vi "Send Message.vi"(6 "ID":string, 8 "error in (no error)":errorcluster, 9 "Data":variant, 10 "Command":string, 11 "RemoteControl.ZMQ in":refnum<class "RemoteControl.ZMQ.lvclass">) -> (0 "error out":errorcluster, 3 "RemoteControl.ZMQ out":refnum<class "RemoteControl.ZMQ.lvclass">)   [LabVIEW 2019, in "RemoteControl.ZMQ.lvlib" / "RemoteControl.ZMQ.lvclass"]
uses:
  RemoteControl.ZMQ.lvclass
  C:/Program Files (x86)/National Instruments/LabVIEW 2019/user.lib/LevyLab/RemoteControl/RemoteControl/RemoteControl.lvclass
  RemoteControl.ZMQ.lvclass/RemoteControl.ZMQ.ctl
  <userlib>/LevyLab/RemoteControl/RemoteControl/RemoteControl.lvclass/RemoteControl.ctl
  <vilib>/PRIrvin/JSON-RPC/JSON-RPC.lvlib
  <vilib>/addons/zeromq/zmq_socket.lvclass
  <userlib>/LevyLab/RemoteControl/RemoteControl/RemoteControl.lvclass
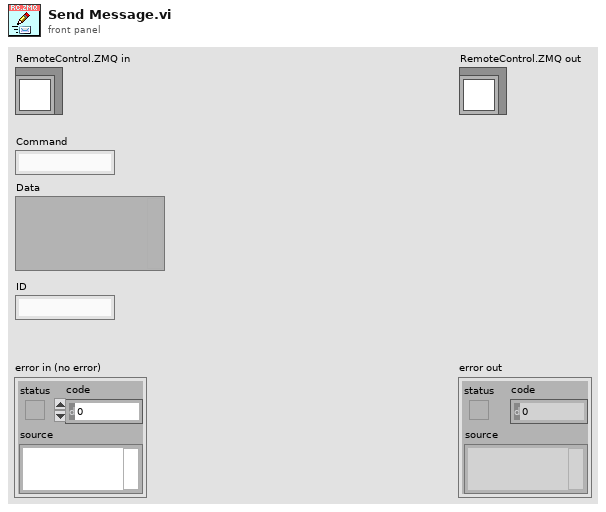
[diagram p1: front panel]
types:
  T1 = typedef "zeromq.lvlib/socket_type.ctl" = enum8{"ZMQ_PAIR", "ZMQ_PUB", "ZMQ_SUB", "ZMQ_REQ", "ZMQ_REP", "ZMQ_DEALER", "ZMQ_ROUTER", "ZMQ_PULL", "ZMQ_PUSH", "ZMQ_XPUB", "ZMQ_XSUB", "ZMQ_STREAM", "ZMQ_SERVER", "ZMQ_CLIENT", "ZMQ_RADIO", "ZMQ_DISH", "ZMQ_GATHER", "ZMQ_SCATTER", "ZMQ_DGRAM"}
  T2 = cluster{"Command":string, "Data":variant, "ID":string}
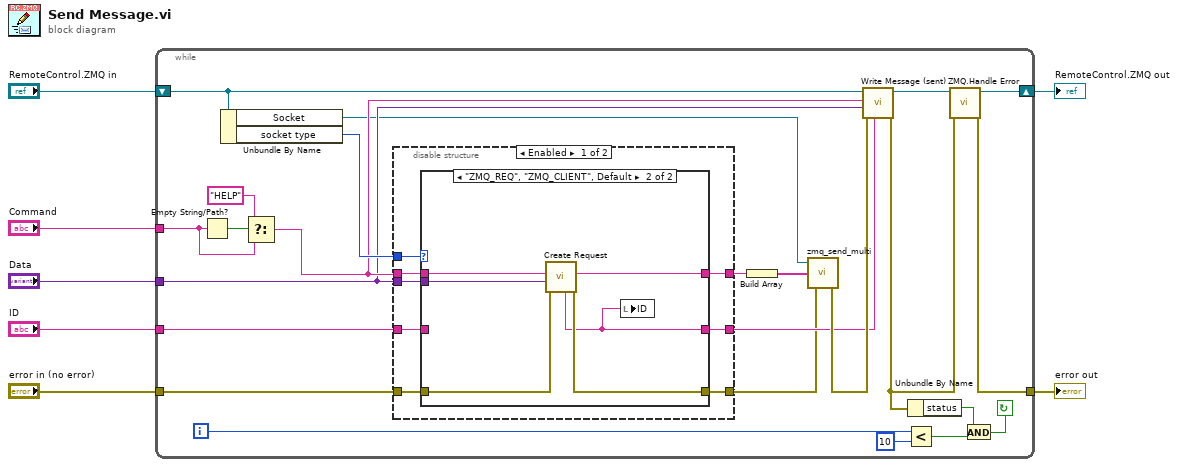
[diagram p0: block diagram]
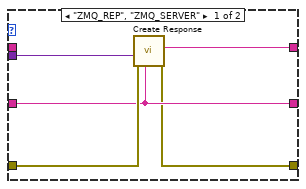
[diagram p2: hidden frame]
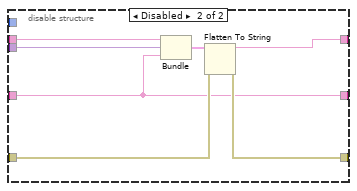
[diagram p3: hidden frame]
diagram:
  n1 = while {
    tunnel: "Command" -> [w15]
    tunnel: "ID" -> [w28]
    tunnel: "Data" -> [w23]
    shift-right: [w17] -> w4
    shift-left: "RemoteControl.ZMQ in" -> [w19]
    tunnel: "error in (no error)" -> [w8]
    tunnel: [w16] -> w3
    i -> [w14]
    stop <- w11 continue-if-true
    n2 = Empty String/Path?(string/path=w15) -> (empty?=w30:bool)
    n3 = Unbundle By Name(w19) -> ("Socket"=w22:refnum<class "zmq_socket.lvclass">, "socket type"=w29:T1)
    n4 = Select(t="HELP", s=w30, f=w15) -> (s? t:f=w27:string)
    n5 = disable-structure shown="Enabled" {
      disable-tunnel: w23 -> [w39 w53]
      disable-tunnel: w27 -> [w38 w54]
      disable-tunnel: [w37 w51] -> w24
      disable-tunnel: w8 -> [w36 w56]
      disable-tunnel: [w35 w55] -> w20
      disable-tunnel: w29 -> [w34 _]
      disable-tunnel: w28 -> [w32 w52]
      disable-tunnel: [w33 w52] -> w25
      frame Enabled {
        n6 = case shown="\"ZMQ_REQ\", \"ZMQ_CLIENT\", Default" w34 {
          tunnel: w38 -> [_ w46]
          tunnel: w39 -> [w40 w47]
          tunnel: [w41 w48] -> w37
          tunnel: w36 -> [w44 w50]
          tunnel: [w42 w49] -> w35
          tunnel: w32 -> [w43 _]
          tunnel: [w43 w45] -> w33
          frame "ZMQ_REP", "ZMQ_SERVER" {
            n7 = call <vilib>:"Create Response.vi"("id"=w43, "error in (no error)"=w44, "result"=w40) -> ("error out"=w42:errorcluster, "<JSON> Response"=w41:string)  [unwired: 7 in]
          }
          frame "ZMQ_REQ", "ZMQ_CLIENT", Default {
            n8 = call <vilib>:"Create Request.vi"("error in (no error)"=w50, "params"=w47, "method"=w46) -> ("error out"=w49:errorcluster, "<JSON> Requests"=w48:string, "IDs"=w45:string)  [unwired: 6 in]
            n9 = local write "ID"(w45) -> ()
          }
        }
      }
      frame Disabled {
        n10 = Bundle("Command"=w54, "Data"=w53, "ID"=w52) -> (w57:T2)  [unwired: 1 in]
        n11 = Flatten To String(anything=w57, error in (no error)=w56) -> (data string=w51:string, error out=w55:errorcluster)  [unwired: 2 in, 1 out]
      }
    }
    n12 = Build Array(w24) -> (w21:string[])
    n13 = call <vilib>:"zmq_send_multi.vi"("error in"=w20, "parts"=w21, "socket in"=w22) -> ("error out"=w26:errorcluster)  [unwired: 1 in, 1 out]
    n14 = call <userlib>:"Write Message (sent).vi"("ID (sent)"=w25, "error in (no error)"=w26, "Data"=w23, "Command (sent)"=w27, "RemoteControl in"=w19) -> ("error out"=w9:errorcluster, "RemoteControl out"=w18:refnum<class "RemoteControl.ZMQ.lvclass">)  [unwired: 5 in]
    n15 = Less?(x=w14, y=10) -> (x < y?=w12:bool)
    n16 = Unbundle By Name(w9) -> ("status"=w10:bool)
    n17 = call "ZMQ.Handle Error.vi"("error in (no error)"=w9, "RemoteControl.ZMQ in"=w18) -> ("error out"=w16:errorcluster, "RemoteControl.ZMQ out"=w17:refnum<class "RemoteControl.ZMQ.lvclass">)  [unwired: 8 in]
    n18 = And(x=w10, y=w12) -> (x .and. y?=w11:bool)
  }
  "error out" <- w3
  "RemoteControl.ZMQ out" <- w4
